vi "Periodic Tasks.vi"(8 "error in":errorcluster) -> ()   [LabVIEW 2019]
doc: "This VI runs in parallel to other tasks. It can contain as many user-defined periodic loops as you need. These can carry out PID or other sorts of timed response."
uses:
  <vilib>/Rock Robotics/WPI/Utilities/WPI_GetSetVariantRefNum.vi
  <vilib>/Rock Robotics/Network Tables/NT Read Boolean.vi
  <vilib>/Rock Robotics/Network Tables/NT Write Number.vi
  Robot Global Data.vi
  <vilib>/Rock Robotics/Network Tables/NT Read Number.vi
  <vilib>/Rock Robotics/WPI/RobotDrive/WPI_RobotDriveArcadeDrive_Standard(NoSaturation).vi
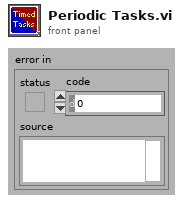
[diagram p1: front panel]
types:
  T1 = typedef "WPI_JoystickDevRef.ctl" = cluster{"Device":T2}
  T2 = typedef "WPI_JoystickDeviceEnum.ctl" = enum16{"USB 0", "USB 1", "USB 2", "USB 3", "USB 4", "USB 5"}
  T3 = typedef "WPI_RobotDriveDevRef.ctl" = cluster{"DevStatus":errorcluster, "Motors[]":T4[], "Square Inputs":bool, "Max Output":dbl}
  T4 = typedef "WPI_MotorControlDeviceRef.ctl" = cluster{"DeviceStatus":errorcluster, "Type":T5, "PWM":cluster{"PWM Channel":T6, "DeadBand":T7}, "CAN":cluster{"Device Number":u8, "SetOutput VI Ref":variant, "GetOutput VI Ref":variant, "Enable VI Ref":variant, "Disable VI Ref":variant, "Data":variant}, "Invert":bool, "DIO PWM":cluster{"PWM \"Enable\" Channel":T6, "DIOChannel":T8, "PWM Rate":dbl}}
  T5 = typedef "WPI_MotorControlType.ctl" = enum16{"PWM", "CAN", "DIO PWM"}
  T6 = typedef "FPGA_DIOPWMChannel.ctl" = enum8{"PWM 0", "PWM 1", "PWM 2", "PWM 3", "PWM 4", "PWM 5", "PWM 6", "PWM 7", "PWM 8", "PWM 9", "PWM MXP 0", "PWM MXP 1", "PWM MXP 2", "PWM MXP 3", "PWM MXP 4", "PWM MXP 5", "PWM MXP 6", "PWM MXP 7", "PWM MXP 8", "PWM MXP 9", "Invalid"}
  T7 = typedef "WPI_PWMDeadband.ctl" = cluster{"Name":string, "maxPositivePwm":i32, "minPositivePwm":i32, "centerPwm":i32, "maxNegativePwm":i32, "minNegativePwm":i32, "angularRange":u16}
  T8 = typedef "FPGA_DIOChannel.ctl" = enum8{"DIO 0", "DIO 1", "DIO 2", "DIO 3", "DIO 4", "DIO 5", "DIO 6", "DIO 7", "DIO 8", "DIO 9", "DIO MXP 0", "DIO MXP 1", "DIO MXP 2", "DIO MXP 3", "DIO MXP 4", "DIO MXP 5", "DIO MXP 6", "DIO MXP 7", "DIO MXP 8", "DIO MXP 9", "DIO MXP 10", "DIO MXP 11", "DIO MXP 12", "DIO MXP 13", "DIO MXP 14", "DIO MXP 15", "SPI Port CS1", "SPI Port CS2", "SPI Port CS3", "SPI Port MISO", "SPI Port MOSI", "Invalid"}
  T9 = cluster{"JoystickDevRef":T1, "RobotDriveDevRef":T3}
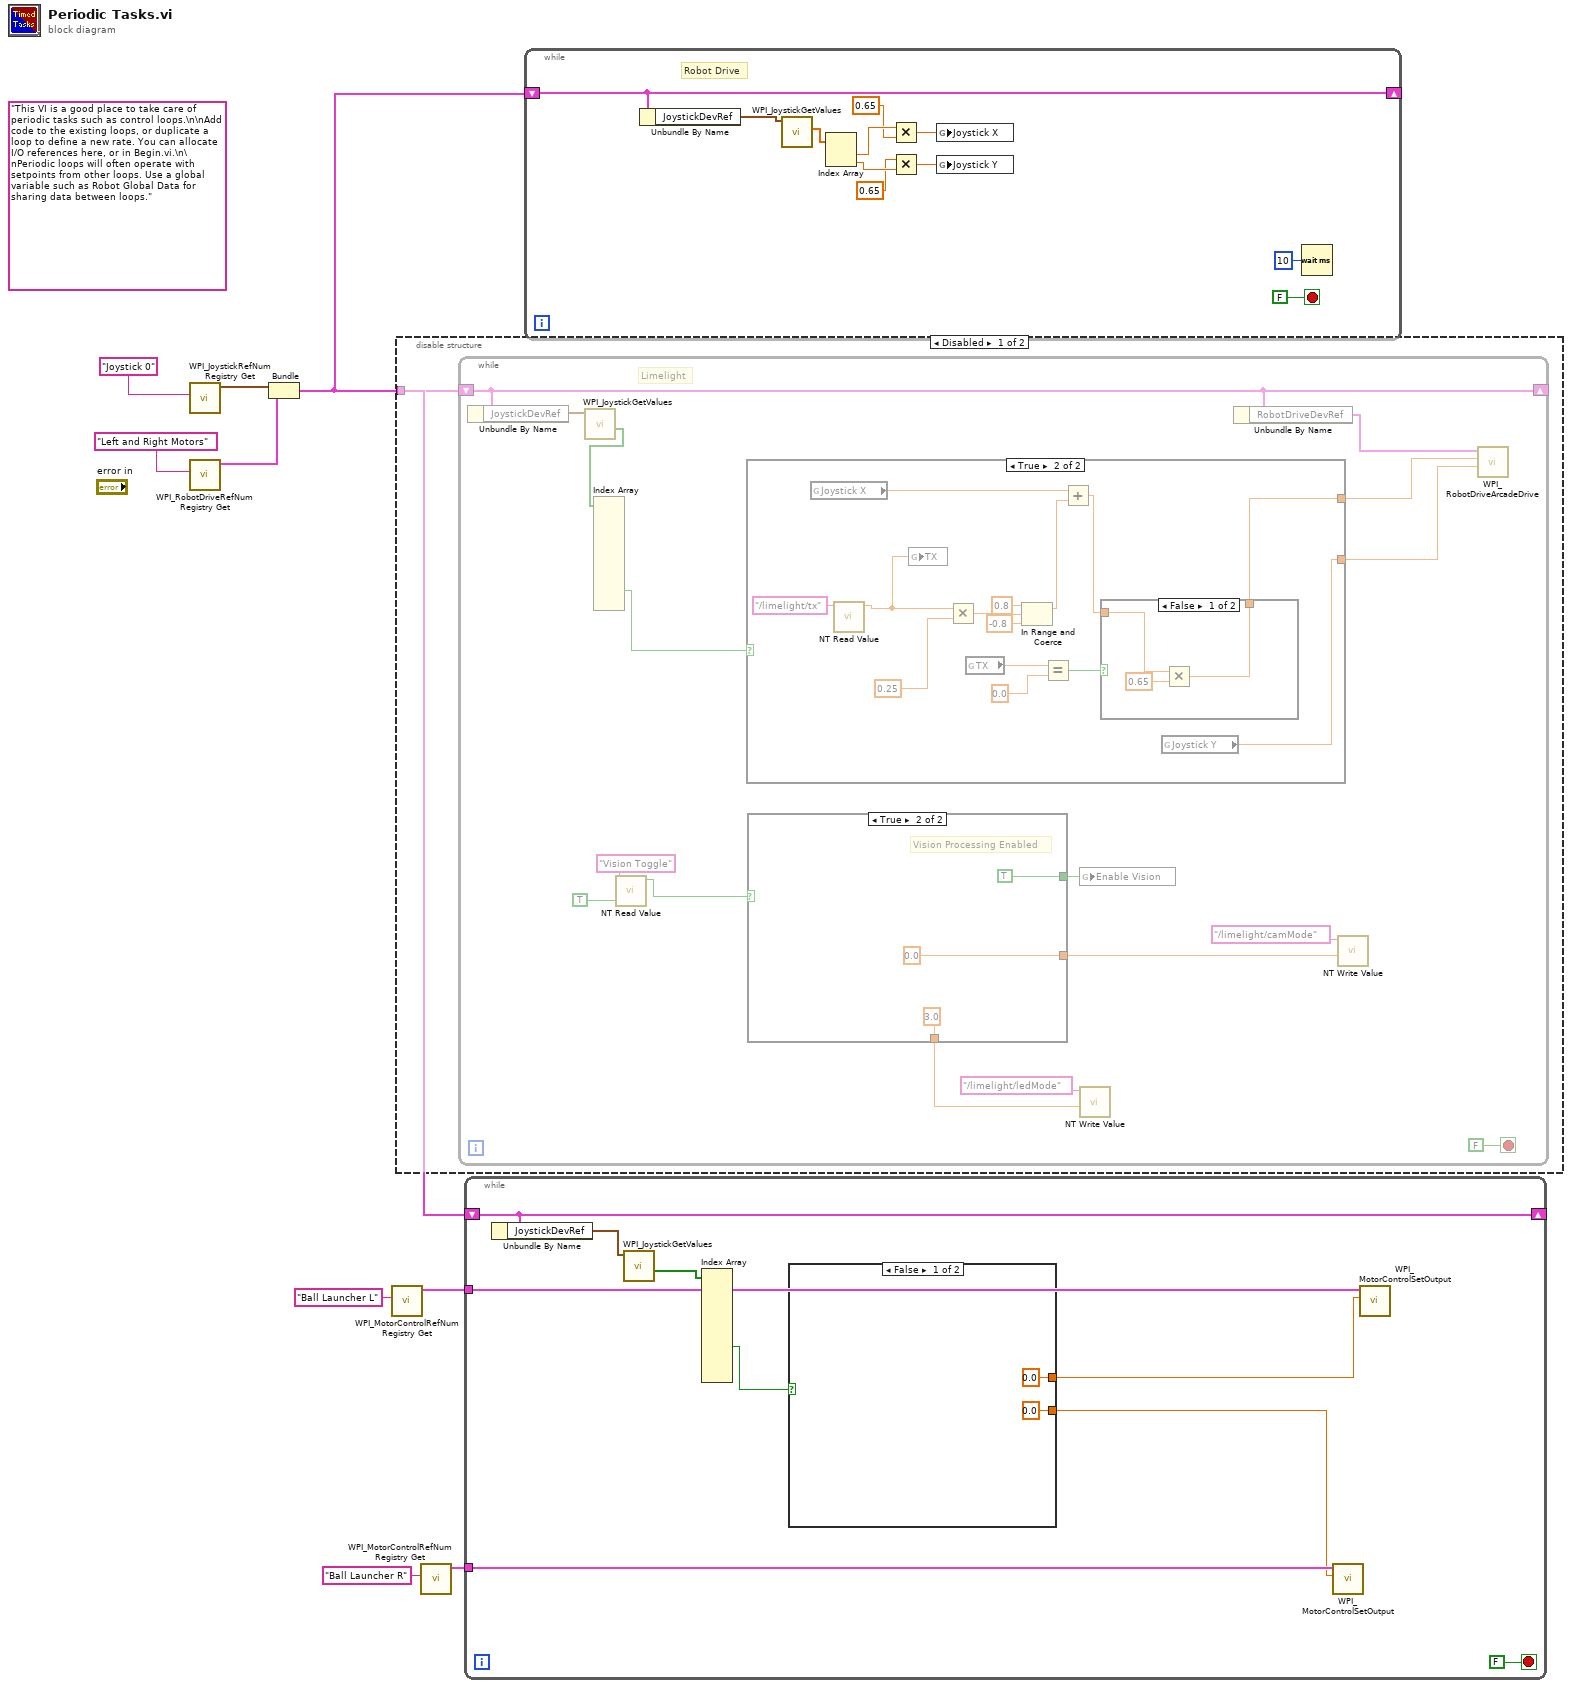
[diagram p0: block diagram]
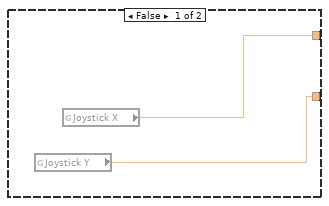
[diagram p2: hidden frame]
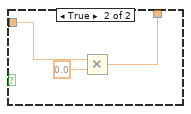
[diagram p3: hidden frame]
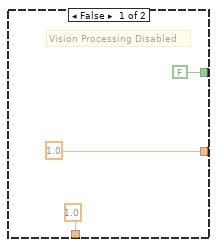
[diagram p4: hidden frame]
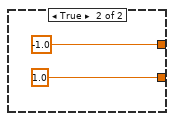
[diagram p6: hidden frame]
diagram:
  (unwired) "This VI is a good place to take care of periodic tasks such as control loops.\n\nAdd code to the existing loops, or duplicate a loop to define a new rate. You can allocate I/O references here, or in Begin.vi.\n\nPeriodic loops will often operate with setpoints from other loops. Use a global variable such as Robot Global Data for sharing data between loops."
  n1 = call <vilib>:"WPI_JoystickRefNum Registry Get.vi"("refnum name"="Joystick 0") -> ("JoystickDevRef"=w7:T1)  [unwired: 1 in, 9 out]
  n2 = call <vilib>:"WPI_RobotDriveRefNum Registry Get.vi"("refnum name"="Left and Right Motors") -> ("RobotDriveDevRef"=w6:T3)  [unwired: 1 in, 9 out]
  n3 = Bundle("JoystickDevRef"=w7, "RobotDriveDevRef"=w6) -> (w3:T9)  [unwired: 1 out]
  n4 = call <vilib>:"WPI_MotorControlRefNum Registry Get.vi"("refnum name"="Ball Launcher L") -> ("MotorControlDevRef"=w4:T4)  [unwired: 9 in, 1 out]
  n5 = disable-structure shown="Disabled" {
    disable-tunnel: w3 -> [w10 _]
    frame Disabled {
      n6 = while {
        shift-right: [w22] -> _
        shift-left: w10 -> [w22]
        stop <- FALSE stop-if-true
        # "Limelight"
        n7 = Unbundle By Name(w22) -> ("JoystickDevRef"=w21:T1)
        n8 = call <vilib>:"WPI_JoystickGetValues.vi"("JoystickDevRef"=w21) -> ("Buttons"=w20:bool[])  [unwired: 6 in, 4 out]
        n9 = Index Array(array=w20) -> (element #10=w14:bool)  [unwired: 12 in, 11 out]
        n10 = call-poly <vilib>:"NT Read Value.vi"("Default Value"=TRUE, "Name"="Vision Toggle") -> ("Boolean"=w13:bool)  [unwired: 8 in, 1 out]
        n11 = case shown="True" w14 {
          tunnel: [w28 w33] -> w23
          tunnel: [w27 w29] -> w11
          frame False {
            n12 = global read "Robot Global Data.vi" "Joystick Y"() -> (w27:dbl)
            n13 = global read "Robot Global Data.vi" "Joystick X"() -> (w28:dbl)
          }
          frame True {
            n14 = global read "Robot Global Data.vi" "Joystick X"() -> (w41:dbl)
            n15 = call-poly <vilib>:"NT Read Value.vi"("Name"="/limelight/tx") -> ("Numeric"=w35:dbl)  [unwired: 9 in, 1 out]
            n16 = global write "Robot Global Data.vi" "TX"(w35) -> ()
            n17 = Multiply(x=w35, y=0.25) -> (x*y=w39:dbl)
            n18 = global read "Robot Global Data.vi" "TX"() -> (w31:dbl)
            n19 = In Range and Coerce(upper limit=0.8, x=w39, lower limit=-0.8) -> (coerced(x)=w40:dbl)  [unwired: 1 out]
            n20 = Equal?(x=w31, y=0.0) -> (x = y?=w32:bool)
            n21 = Add(x=w41, y=w40) -> (x+y=w34:dbl)
            n22 = case shown="False" w32 {
              tunnel: w34 -> [w44 w48]
              tunnel: [w45 w46] -> w33
              frame False {
                n23 = Multiply(x=w44, y=0.65) -> (x*y=w45:dbl)
              }
              frame True {
                n24 = Multiply(x=w48, y=0.0) -> (x*y=w46:dbl)
              }
            }
            n25 = global read "Robot Global Data.vi" "Joystick Y"() -> (w29:dbl)
          }
        }
        n26 = case shown="True" w13 {
          tunnel: [FALSE ("Enable Vision") TRUE ("Enable Vision")] -> w25
          tunnel: [1.0 ("Numeric") 0.0 ("Numeric")] -> w18
          tunnel: [1.0 ("Numeric") 3.0 ("Numeric")] -> w15
          frame False {
            # "Vision Processing Disabled"
          }
          frame True {
            # "Vision Processing Enabled"
          }
        }
        n27 = global write "Robot Global Data.vi" "Enable Vision"(w25) -> ()
        n28 = call-poly <vilib>:"NT Write Value.vi"("Numeric"=w15, "Name"="/limelight/ledMode") -> ()  [unwired: 9 in, 1 out]
        n29 = Unbundle By Name(w22) -> ("RobotDriveDevRef"=w24:T3)
        n30 = call-poly <vilib>:"NT Write Value.vi"("Numeric"=w18, "Name"="/limelight/camMode") -> ()  [unwired: 9 in, 1 out]
        n31 = call-poly <vilib>:"WPI_RobotDriveArcadeDrive.vi"("Y axis value"=w11, "X axis value"=w23, "RobotDriveDevRef"=w24) -> ()  [unwired: 6 in, 3 out]
      }
    }
    frame Enabled {
    }
  }
  n32 = call <vilib>:"WPI_MotorControlRefNum Registry Get.vi"("refnum name"="Ball Launcher R") -> ("MotorControlDevRef"=w1:T4)  [unwired: 9 in, 1 out]
  n33 = while {
    tunnel: w4 -> [w62]
    shift-right: [w61] -> _
    shift-left: w3 -> [w61]
    tunnel: w1 -> [w56]
    stop <- FALSE stop-if-true
    n34 = Unbundle By Name(w61) -> ("JoystickDevRef"=w60:T1)
    n35 = call <vilib>:"WPI_JoystickGetValues.vi"("JoystickDevRef"=w60) -> ("Buttons"=w59:bool[])  [unwired: 6 in, 4 out]
    n36 = Index Array(array=w59) -> (element #8=w58:bool)  [unwired: 12 in, 11 out]
    n37 = case shown="False" w58 {
      tunnel: [0.0 ("Output") -1.0 ("Output")] -> w57
      tunnel: [0.0 ("Output") 1.0 ("Output")] -> w55
      frame False {
      }
      frame True {
      }
    }
    n38 = call <vilib>:"WPI_MotorControlSetOutput.vi"("Output"=w55, "MotorControlDevRef"=w56) -> ()  [unwired: 7 in, 3 out]
    n39 = call <vilib>:"WPI_MotorControlSetOutput.vi"("Output"=w57, "MotorControlDevRef"=w62) -> ()  [unwired: 7 in, 3 out]
  }
  n40 = while {
    shift-right: [w77] -> _
    shift-left: w3 -> [w77]
    stop <- FALSE stop-if-true
    # "Robot Drive"
    n41 = Unbundle By Name(w77) -> ("JoystickDevRef"=w75:T1)
    n42 = call <vilib>:"WPI_JoystickGetValues.vi"("JoystickDevRef"=w75) -> ("Axes"=w74:dbl[])  [unwired: 6 in, 4 out]
    n43 = Index Array(array=w74) -> (element #1=w73:dbl, element #2=w71:dbl)  [unwired: 2 in]
    n44 = Multiply(x=w73, y=0.65) -> (x*y=w69:dbl)
    n45 = Multiply(x=0.65, y=w71) -> (x*y=w68:dbl)
    n46 = global write "Robot Global Data.vi" "Joystick X"(w69) -> ()
    n47 = global write "Robot Global Data.vi" "Joystick Y"(w68) -> ()
    n48 = Wait (ms)(milliseconds to wait=u32 10) -> ()  [unwired: 1 out]
  }
